vi "H5Pget_small_data_block_size.vi"(6 "error in (no error)":errorcluster, 9 "HDF5 Property Ref":T1) -> (0 "error out":errorcluster, 2 "Size":u64=2048, 3 "HDF5 Ref out":T1)   [LabVIEW 2017]
doc: "Retrieves the current small data block size setting."
uses:
  <vilib>/UPVI/lvhdf5/library.llb/HDF5 Ref.ctl
  <vilib>/UPVI/lvhdf5/hdf5.dll
panel:
  # "LVHDF5 Toolkit\nCopyright (c) 2005-2013 by Jason D. Sommerville\nCopyright (c) 2014 by UPVI, LLC.\n\nThis use and distribution of this file is governed by the terms found in \nLICENSE.txt distributed with this toolkit and installed at\n <user.lib>\\_lvhdf5\\LICENSE.txt"
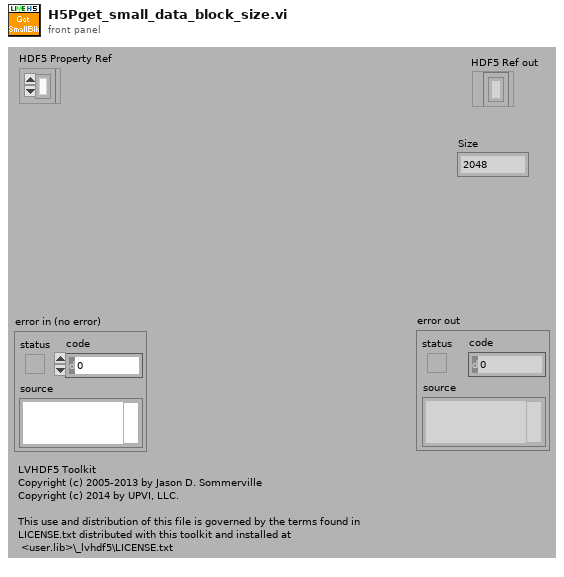
[diagram p1: front panel]
types:
  T1 = typedef "HDF5 Ref.ctl" = refnum<k1>
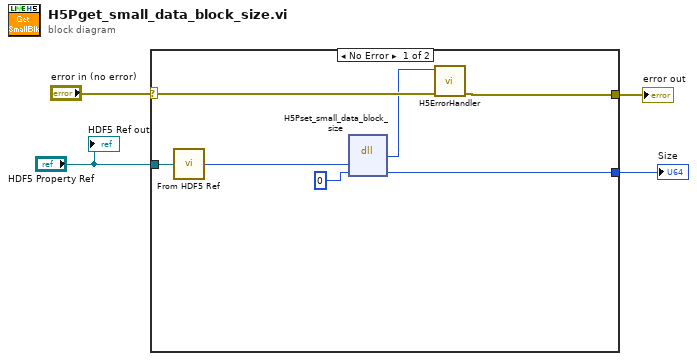
[diagram p0: block diagram]
diagram:
  n1 = case shown="No Error" "error in (no error)" {
    selector: "error in (no error)" -> [w11 w12]
    tunnel: [w6 w12] -> w3
    tunnel: "HDF5 Property Ref" -> [w9 _]
    tunnel: [w5 _] -> w1
    frame No Error {
      n2 = call <vilib>:"From HDF5 Ref.vi"("HDF5 Ref"=w9) -> ("I32"=w8:i32)
      n3 = dll-call lib="C:/Program Files/National Instruments/LabVIEW 2017/vi.lib/UPVI/lvhdf5/hdf5.dll" fn="H5Pset_small_data_block_size"("plist_id"=w8, "size"=u64 0) -> ("return type"=w10:i32, "size"=w5:u64)  [unwired: 4 in, 2 out]
      n4 = call <vilib>:"H5ErrorHandler.vi"("error in (no error)"=w11, "herr_t"=w10) -> ("error out"=w6:errorcluster)  [unwired: 3 in, 4 out]
    }
    frame Error {
    }
  }
  "error out" <- w3
  "Size" <- w1
  "HDF5 Ref out" <- "HDF5 Property Ref"
